vi "HTTPMethod 2.vi"(7 "LabVIEW Web Service Request":refnum<class "Web Request.lvclass">) -> ()   [LabVIEW 2018]
uses:
  <vilib>/wsapi/Web Request.lvclass
  <vilib>/JDP Science/JSONtext/support/Format JSON Object.vi
  <vilib>/JDP Science/JDP Science Common Utilities/Timestamp/JDP Timestamp.lvlib
  <userlib>/_OpenG.lib/string/string.llb/openg_string.lvlib
  <vilib>/JDP Science/JSONtext/JSONtext.lvlib
panel:
  out "zadanie 2":string
  out "jazda 2":string caption="<JSON>Object"
  out "error out 6":errorcluster
  out "error out 5":errorcluster
  out "JSON Error out 2":errorcluster
  out "error out 4":errorcluster
  in  "LabVIEW Web Service Request 2":refnum<class "Web Request.lvclass">
  out "error out 2":errorcluster
  out "error out":errorcluster
  # "Use the Web Service Request input terminal to call the VIs on the Web Services palette. Do not remove it from the connector pane unless you don't need access to the palette."
  # "Each additional control wired to the connector pane will be available as an input in the URL. To include an indicator in terminal-mode output (the default setting), it must also be wired to the connector pane."
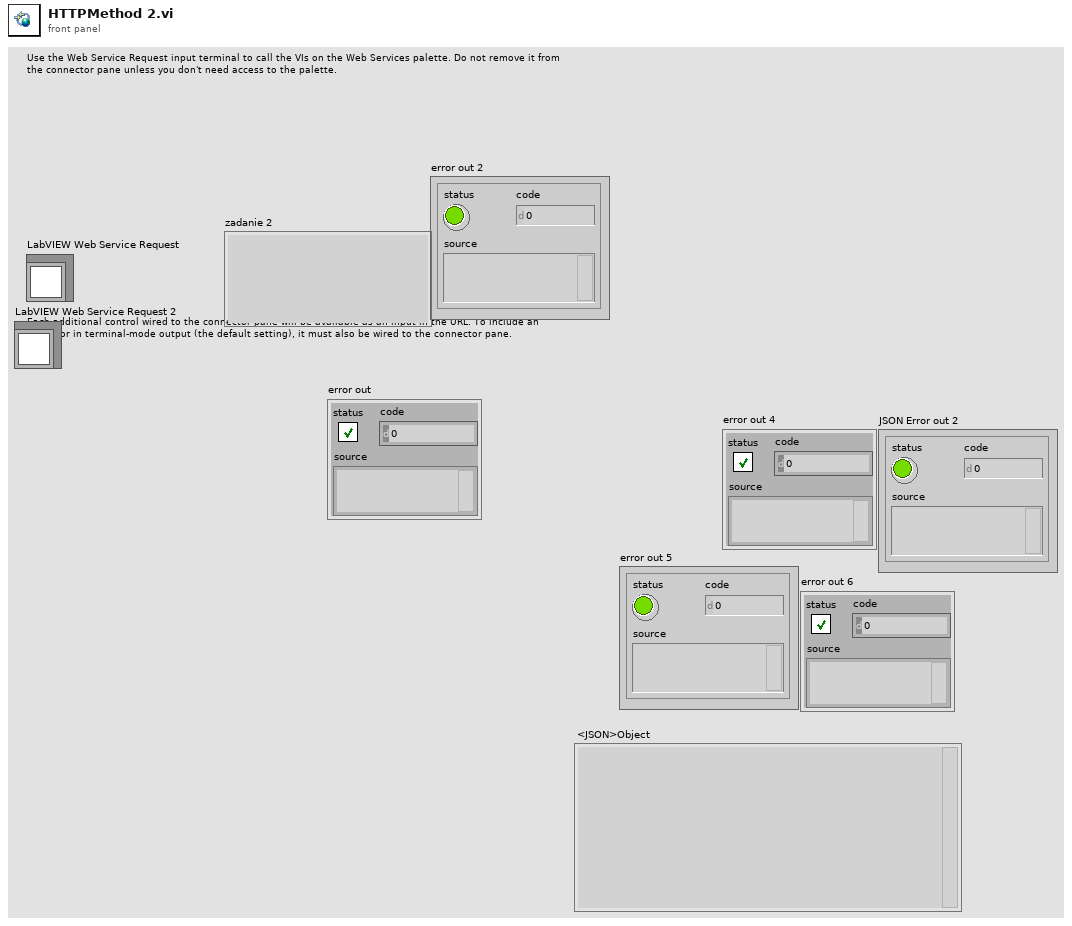
[diagram p1: front panel]
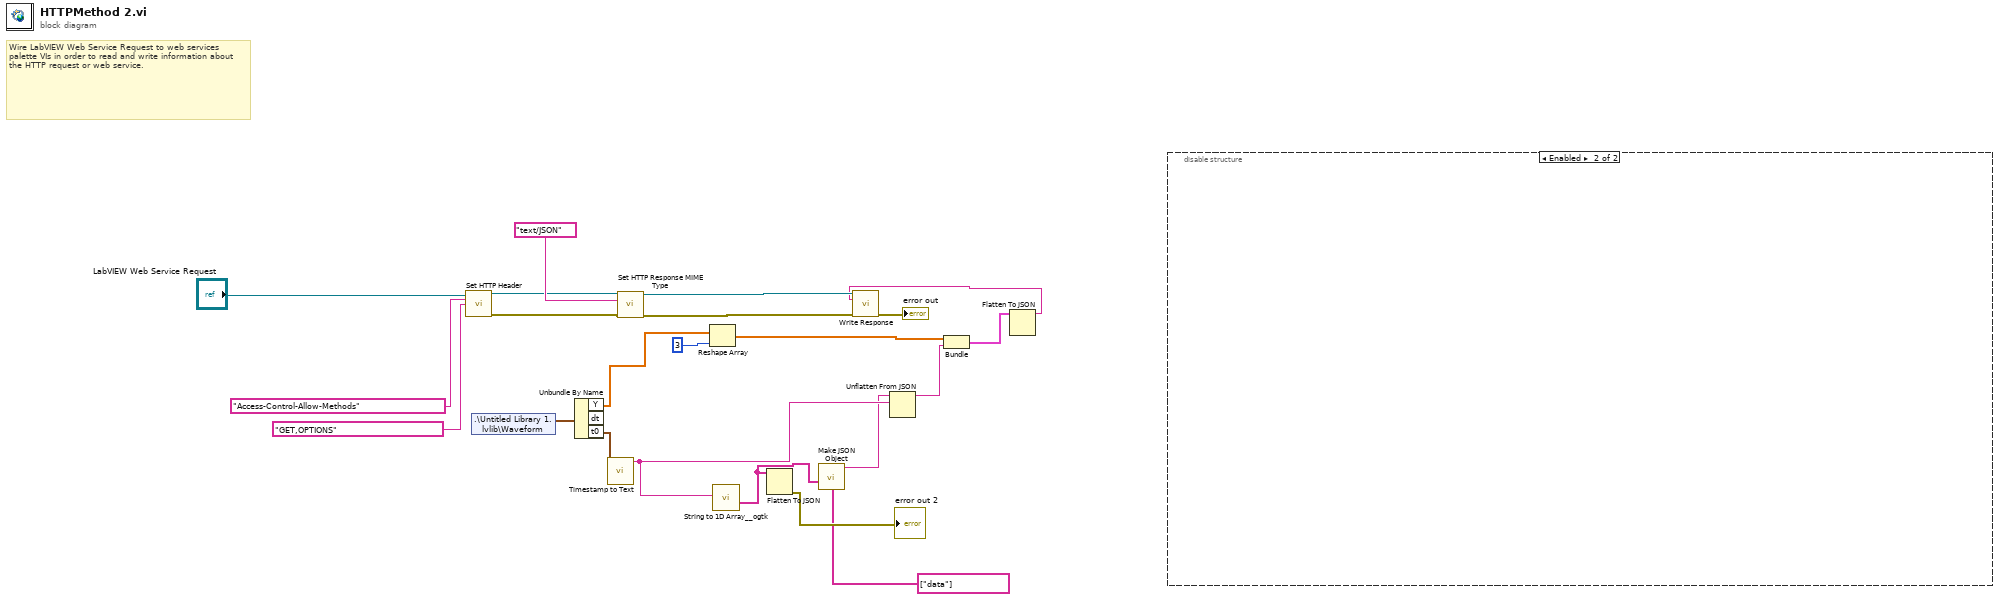
[diagram p0: block diagram]
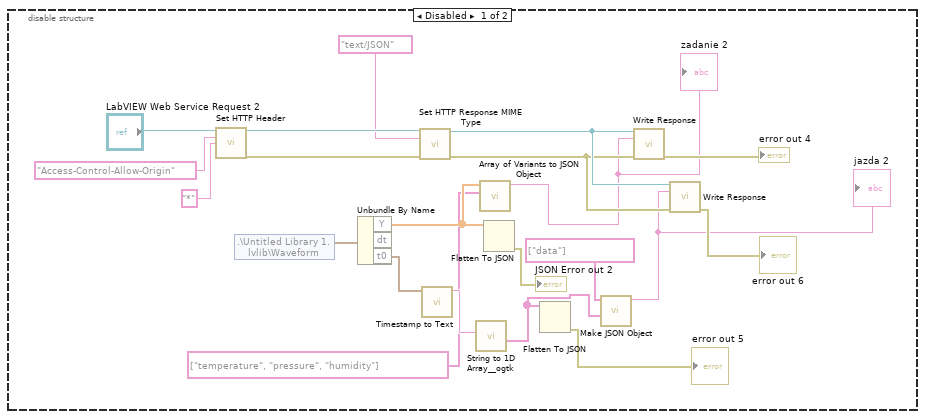
[diagram p2: hidden frame]
diagram:
  # "Wire LabVIEW Web Service Request to web services palette VIs in order to read and write information about the HTTP request or web service."
  n1 = call <vilib>:"Set HTTP Header.vi"("LabVIEW Web Service Request"="LabVIEW Web Service Request", "header"="Access-Control-Allow-Methods", "header value"="GET,OPTIONS") -> ("LabVIEW Web Service Request out"=w5:refnum<class "Web Request.lvclass">, "error out"=w4:errorcluster)  [unwired: 11 in]
  n2 = shared-variable ".\\Untitled Library 1.lvlib\\Waveform"() -> (w21:waveform(dbl))  [unwired: 1 in, 1 out]
  n3 = Unbundle By Name(w21) -> ("Y"=w9:dbl[], "t0"=w15:timestamp)  [unwired: 1 out]
  n4 = call <vilib>:"Timestamp to Text.vi"("Time Stamp"=w15) -> ("Timestamp (RFC3339)"=w13:string)  [unwired: 9 in, 1 out]
  n5 = call <vilib>:"Set HTTP Response MIME Type.vi"("LabVIEW Web Service Request"=w5, "MIME type (text/html)"="text/JSON", "error in (no error)"=w4) -> ("LabVIEW Web Service Request out"=w17:refnum<class "Web Request.lvclass">, "error out"=w16:errorcluster)  [unwired: 11 in]
  n6 = Reshape Array(w9, 3 ("dimension size")) -> (w6:dbl[])
  n7 = call <userlib>:"String to 1D Array__ogtk.vi"("string"=w13) -> ("Array of Strings"=w19:string[])  [unwired: 10 in]
  n8 = Flatten To JSON(anything=w19) -> (11:→"error out 2":errorcluster)  [unwired: 2 in, 1 out]
  n9 = call <vilib>:"Make JSON Object.vi"("JSON Items"=w19, "Item Names"=string[] ["data"]) -> ("<JSON>"=w12:string)  [unwired: 8 in, 1 out]
  n10 = Unflatten From JSON(JSON string=w12, type and defaults=w13) -> (value=w8:string)  [unwired: 5 in, 1 out]
  n11 = Bundle("Y"=w6, "Timestamp (RFC3339)"=w8) -> (w7:cluster{"Y":dbl[], "Timestamp (RFC3339)":string})  [unwired: 1 in]
  n12 = Flatten To JSON(anything=w7) -> (JSON string=w11:string)  [unwired: 2 in, 1 out]
  n13 = call <vilib>:"Write Response.vi"("LabVIEW Web Service Request"=w17, "response string"=w11, "error in (no error)"=w16) -> ("error out"=→"error out":errorcluster)  [unwired: 11 in, 1 out]
  n14 = disable-structure shown="Enabled" {
    frame Disabled {
      n15 = call <vilib>:"Set HTTP Header.vi"("LabVIEW Web Service Request"="LabVIEW Web Service Request 2", "header"="Access-Control-Allow-Origin", "header value"="*") -> ("LabVIEW Web Service Request out"=w40:refnum<class "Web Request.lvclass">, "error out"=w39:errorcluster)  [unwired: 11 in]
      n16 = shared-variable ".\\Untitled Library 1.lvlib\\Waveform"() -> (w35:waveform(dbl))  [unwired: 1 in, 1 out]
      n17 = Unbundle By Name(w35) -> ("Y"=w26:dbl[], "t0"=w34:timestamp)  [unwired: 1 out]
      n18 = call <vilib>:"Set HTTP Response MIME Type.vi"("LabVIEW Web Service Request"=w40, "MIME type (text/html)"="text/JSON", "error in (no error)"=w39) -> ("LabVIEW Web Service Request out"=w32:refnum<class "Web Request.lvclass">, "error out"=w31:errorcluster)  [unwired: 11 in]
      n19 = call <vilib>:"Timestamp to Text.vi"("Time Stamp"=w34) -> ("Timestamp (RFC3339)"=w33:string)  [unwired: 9 in, 1 out]
      n20 = call <userlib>:"String to 1D Array__ogtk.vi"("string"=w33) -> ("Array of Strings"=w28:string[])  [unwired: 10 in]
      n21 = call <vilib>:"Array of Variants to JSON Object.vi"("Names"=string[] ["temperature", "pressure", "humidity"], "Array"=w26) -> ("<JSON>"=w23:string)  [unwired: 8 in, 1 out]
      "zadanie 2" <- w23
      n22 = Flatten To JSON(anything=w26) -> (11:→"JSON Error out 2":errorcluster)  [unwired: 2 in, 1 out]
      n23 = Flatten To JSON(anything=w28) -> (11:→"error out 5":errorcluster)  [unwired: 2 in, 1 out]
      n24 = call <vilib>:"Make JSON Object.vi"("JSON Items"=w28, "Item Names"=string[] ["data"]) -> ("<JSON>"=w24:string)  [unwired: 8 in, 1 out]
      "jazda 2" <- w24
      n25 = call <vilib>:"Write Response.vi"("LabVIEW Web Service Request"=w32, "response string"=w23, "error in (no error)"=w31) -> ("error out"=→"error out 4":errorcluster)  [unwired: 11 in, 1 out]
      n26 = call <vilib>:"Write Response.vi"("LabVIEW Web Service Request"=w32, "response string"=w24, "error in (no error)"=w31) -> ("error out"=→"error out 6":errorcluster)  [unwired: 11 in, 1 out]
    }
    frame Enabled {
    }
  }
